vi "Pusher_ClientExample.vi"() -> ()   [LabVIEW 2009]
uses:
  public/Pusher_Client_MonitorData.ctl
  Client.lvclass
panel:
  in  "Channel":string="LvChannel"
  in  "api_key":string
  out "PingPong":i32
  in  "_data":T1
  out "Received Data":string
  in  "stop":bool
  # "Instructions:\n1- Fill in your pusher API key\n2- Run the VI\n3- Use \"Event Creator\" tab on pusher.com to send events \nto your channel in the following format\n\nChannel Name: LvChannel\nEvent name: message\nEvent data: {\"name\":\"joe\",\"age\":\"30\"}"
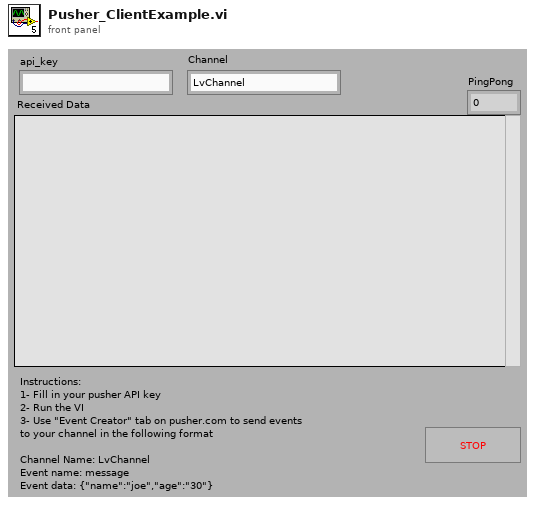
[diagram p1: front panel]
types:
  T1 = typedef "Client.lvclass/Pusher_Client_MonitorData.ctl" = cluster{"EventRef":refnum<user-event>, "EvtRegRef":refnum<event-registration>}
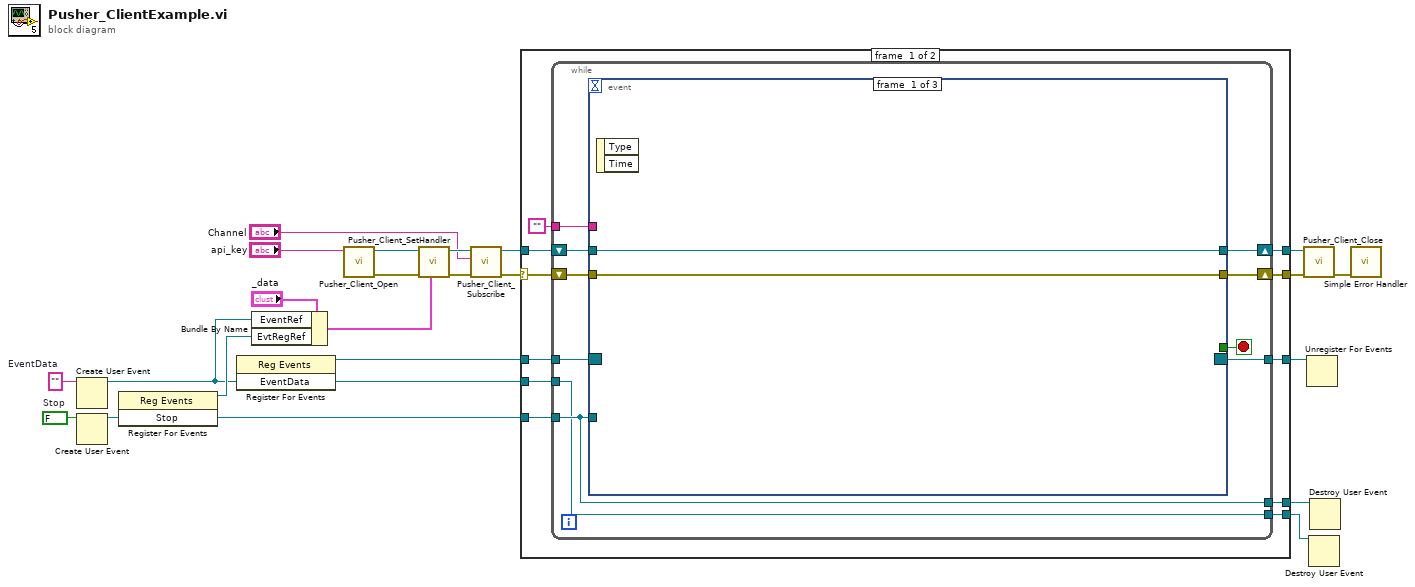
[diagram p0: block diagram]
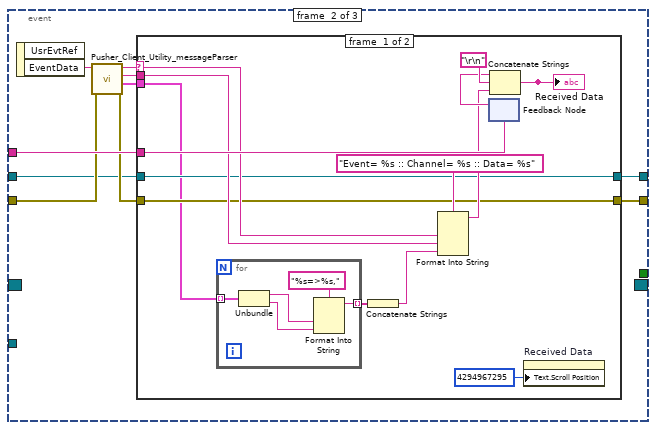
[diagram p2: hidden frame]
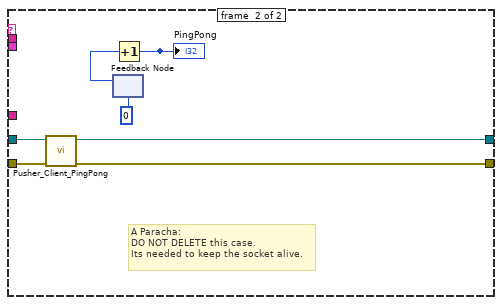
[diagram p3: hidden frame]
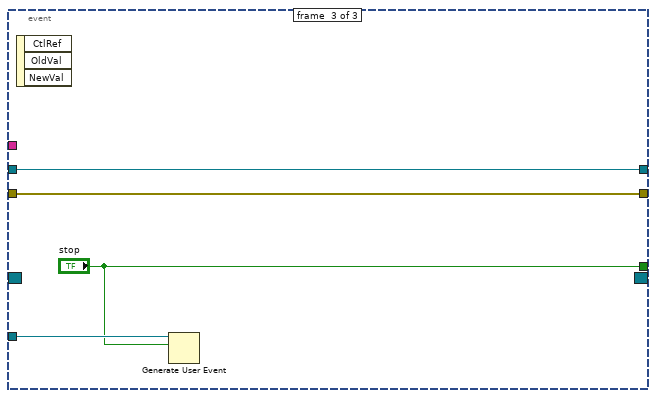
[diagram p4: hidden frame]
diagram:
  w19 = FALSE  # Stop
  w20 = ""  # EventData
  n1 = Create User Event(user event datatype=w20) -> (user event=w13:refnum<user-event>)  [unwired: 1 in, 1 out]
  n2 = Create User Event(user event datatype=w19) -> (user event=w16:refnum<user-event>)  [unwired: 1 in, 1 out]
  n3 = register-events(w16) -> (reference out=w17:refnum<event-registration>)  [unwired: 2 in, 1 out]
  n4 = register-events(w13) -> (reference out=w15:refnum<event-registration>)  [unwired: 2 in, 1 out]
  n5 = Bundle By Name(cluster="_data", "EventRef"=w13, "EvtRegRef"=w17) -> (w5:T1)
  n6 = call "Pusher_Client_Open.vi"("api_key"="api_key") -> ("ErrOut"=w9:errorcluster, "Client out"=w8:refnum<class "Client.lvclass">)  [unwired: 9 in]
  n7 = call "Pusher_Client_SetHandler.vi"("_data"=w5, "ErrIn"=w9, "Client in"=w8) -> ("ErrOut"=w7:errorcluster, "Client out"=w6:refnum<class "Client.lvclass">)  [unwired: 6 in, 1 out]
  n8 = call "Pusher_Client_Subscribe.vi"("ErrIn"=w7, "ChannelName"="Channel", "Client in"=w6) -> ("ErrOut"=w3:errorcluster, "Client out"=w10:refnum<class "Client.lvclass">)  [unwired: 7 in]
  n9 = case shown="No Error" w3 {
    selector: w3 -> [w25 w88]
    tunnel: w16 -> [w33 w87]
    tunnel: w15 -> [w32 w90]
    tunnel: [w31 w90] -> w14
    tunnel: w13 -> [w30 w86]
    tunnel: [w29 w89] -> w12
    tunnel: [w28 w88] -> w11
    tunnel: w10 -> [w26 w89]
    tunnel: [w24 w87] -> w2
    tunnel: [w23 w86] -> w1
    frame #0 {
      n10 = while {
        tunnel: w33 -> [w35]
        tunnel: w32 -> [w43]
        tunnel: [w41] -> w31
        tunnel: w30 -> [w34]
        shift-right: [w38] -> w28
        shift-left: w25 -> [w39]
        shift-right: [w37] -> w29
        shift-left: w26 -> [w40]
        tunnel: "" -> [w36]
        tunnel: [w35] -> w24
        tunnel: [w34] -> w23
        stop <- w42 stop-if-true
        n11 = event shown="[1] <EventData>: User Event" {
          selector: w43 -> [_ _ _]
          dyn-events: [_ _ _] -> w41
          timeout: _ -> [_ _ _]
          tunnel: w35 -> [_ _ w85]
          tunnel: [_ _ "stop"] -> w42
          tunnel: w40 -> [w45 w50 w82]
          tunnel: w39 -> [w44 w53 w83]
          tunnel: [w44 w48 w83] -> w38
          tunnel: [w45 w49 w82] -> w37
          tunnel: w36 -> [_ w55 _]
          event #0 {
            n12 = event-data() -> ()  [unwired: 1 in, 2 out]
          }
          event #1 {
            n13 = event-data() -> ("EventData"=w54:string)  [unwired: 1 in, 1 out]
            n14 = call "Pusher_Client_Utility_messageParser.vi"("ErrIn"=w53, "message"=w54) -> ("ErrOut"=w51:errorcluster, "data"=w46:cluster{"name":string, "value":string}[], "Channel"=w47:string, "Event"=w52:string)  [unwired: 5 in, 1 out]
            n15 = case shown="\"False\", Default" w52 {
              selector: w52 -> [w65 _]
              tunnel: w55 -> [w68 _]
              tunnel: w51 -> [w61 w81]
              tunnel: w50 -> [w60 w80]
              tunnel: [w60 w79] -> w49
              tunnel: [w61 w78] -> w48
              tunnel: w47 -> [w64 _]
              tunnel: w46 -> [w59 _]
              frame #0 {
                n16 = for {
                  tunnel: w59 -> [w74] mode=indexing
                  tunnel: [w70] -> w58 mode=indexing
                  n17 = Unbundle(w74) -> ("name"=w72:string, "value"=w71:string)
                  n18 = Format Into String(format string="%s=>%s,", w72, w71) -> (resulting string=w70:string)  [unwired: 2 in, 1 out]
                }
                n19 = Concatenate Strings(w58) -> (w57:string)
                n20 = Format Into String(format string="Event= %s :: Channel= %s :: Data= %s", w65, w64, w57) -> (resulting string=w62:string)  [unwired: 2 in, 1 out]
                n21 = feedback #1(w68) -> (w66:string)
                n22 = Concatenate Strings(w66, "\r\n", w62) -> (w67:string)
                "Received Data" <- w67
                n23 = property on="Received Data" class="Str"("Text.Scroll Position"=u32 4294967295) -> ()  [unwired: 2 in, 2 out]
              }
              frame #1 {
                # "A Paracha:\nDO NOT DELETE this case.\nIts needed to keep the socket alive."
                n24 = call "Pusher_Client_PingPong.vi"("ErrIn"=w81, "Client in"=w80) -> ("ErrOut"=w78:errorcluster, "Client out"=w79:refnum<class "Client.lvclass">)  [unwired: 8 in]
                n25 = feedback #2(0) -> (w76:i32)
                n26 = Increment(x=w76) -> (x+1=w75:i32)
                "PingPong" <- w75
              }
            }
          }
          event #2 {
            n27 = event-data() -> ()  [unwired: 1 in, 3 out]
            n28 = Generate User Event(user event=w85, event data cluster="stop") -> ()  [unwired: 1 in, 2 out]
          }
        }
      }
    }
    frame #1 {
    }
  }
  n29 = call "Pusher_Client_Close.vi"("ErrIn"=w11, "Client in"=w12) -> ("ErrOut"=w21:errorcluster)  [unwired: 9 in]
  n30 = Unregister For Events(event registration refnum=w14) -> ()  [unwired: 1 in, 1 out]
  n31 = Destroy User Event(user event=w1) -> ()  [unwired: 1 in, 1 out]
  n32 = Destroy User Event(user event=w2) -> ()  [unwired: 1 in, 1 out]
  n33 = call <vilib>:"Simple Error Handler.vi"("error in (no error)"=w21) -> ()  [unwired: 4 in, 5 out]
